vi "Save File Find the Headers and Fix Array.vi"(8 "Error In":errorcluster, 11 "Input":string[][](array[string])) -> (0 "Error Out":errorcluster, 3 "Output":string[][](array[string]))   [LabVIEW 2016]
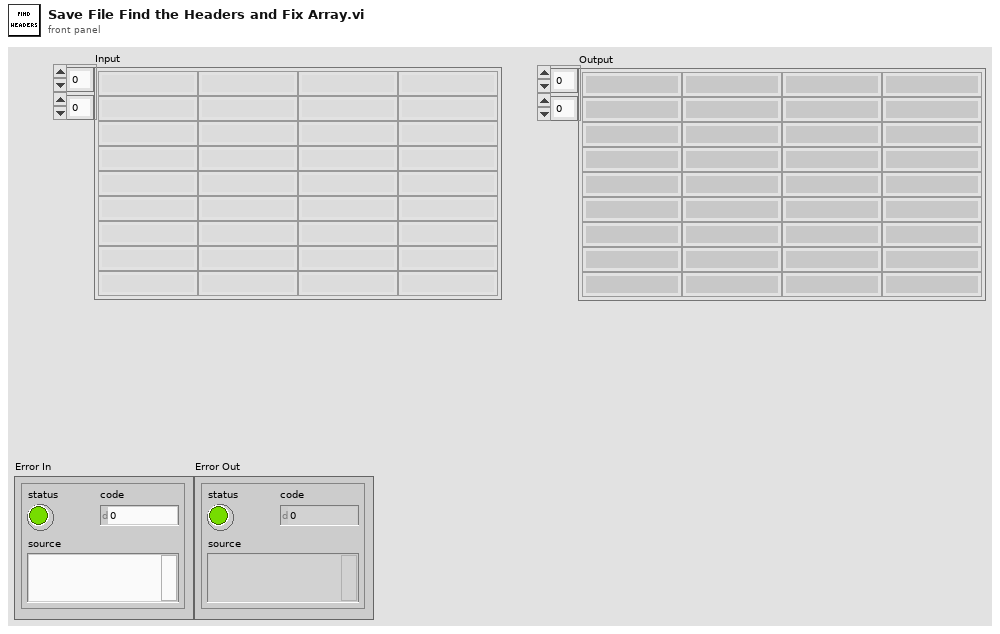
[diagram p1: front panel]
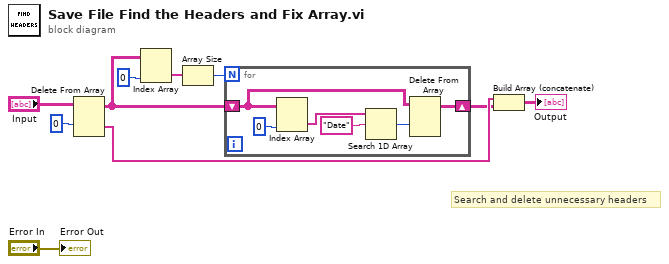
[diagram p0: block diagram]
diagram:
  # "Search and delete unnecessary headers"
  n1 = Delete From Array(array="Input", index (row)=0) -> (deleted portion=w9:string[], array with subset deleted=w5:string[][])  [unwired: 2 in]
  n2 = Index Array(array=w5, index (col)=0 ("disabled index (col)")) -> (element=w6:string[])  [unwired: 1 in]
  n3 = Array Size(array=w6) -> (size(s)=w7:i32)
  n4 = for {
    N: w7 -> [_]
    shift-right: [w16] -> w8
    shift-left: w5 -> [w13]
    n5 = Index Array(array=w13, index (col)=0 ("disabled index (col)")) -> (element=w11:string[])  [unwired: 1 in]
    n6 = Search 1D Array(1D array=w11, element="Date" ("y")) -> (index of element=w14:i32)  [unwired: 1 in]
    n7 = Delete From Array(array=w13, index (row)=w14) -> (array with subset deleted=w16:string[][])  [unwired: 2 in, 1 out]
  }
  n8 = Build Array (concatenate)(w9, w8) -> (→"Output":string[][])
  "Error Out" <- "Error In"
